vi "Receive Value.vi"(10 "Numeric":dbl, 11 "Caller in":refnum<class "Caller B.lvclass">) -> (3 "Caller out":refnum<class "Caller B.lvclass">)   [LabVIEW 2023, in "Caller B.lvlib" / "Caller B.lvclass"]
uses:
  Caller B.lvclass
  Caller B.lvclass/Caller B.ctl
  Localization.vi
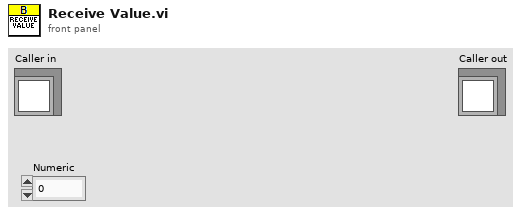
[diagram p1: front panel]
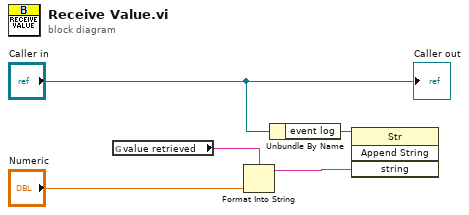
[diagram p0: block diagram]
diagram:
  n1 = global read "Localization.vi" "value retrieved"() -> (w2:string)
  n2 = Format Into String(format string=w2, "Numeric") -> (resulting string=w1:string)  [unwired: 2 in, 1 out]
  n3 = Unbundle By Name("Caller in") -> ("event log"=w3:refnum<vi>)
  n4 = invoke on="Invoke Node" class="Str" method="Append String"(reference=w3, "string"=w1) -> ()  [unwired: 2 in, 4 out]
  "Caller out" <- "Caller in"
